vi "Process_Rect.vi"(10 "Image to process":T2, 11 "Difference image":T2) -> (0 "Target Dist":dbl, 1 "Vertical Angle":dbl, 2 "Horizontal Angle":dbl, 3 "Processed Image Out":T2, 4 "Bounding Rect":T1, 5 "Found Target":bool)   [LabVIEW 2012]
uses:
  <vilib>/vision/Image Controls.llb/IMAQ Image.ctl
  <vilib>/vision/NI_Vision_Development_Module.lvlib
panel:
  in  "Vertical Angle Offset":dbl=4.39
  out "dt 2":u32
  out "dt 1":u32
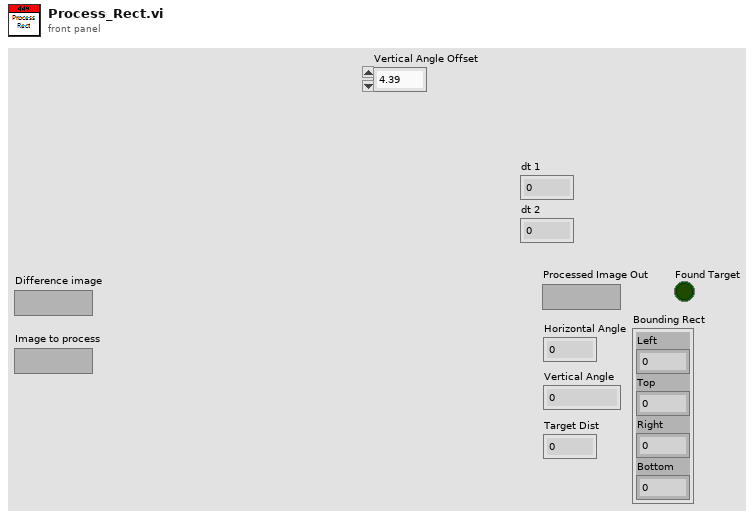
[diagram p1: front panel]
types:
  T1 = cluster{"Left":dbl, "Top":dbl, "Right":dbl, "Bottom":dbl}
  T2 = typedef "IMAQ Image.ctl" = refnum<image>
  T3 = cluster{"Area":dbl, "Number of Holes":dbl, "Bounding Rect":cluster{"Left":dbl, "Top":dbl, "Right":dbl, "Bottom":dbl}, "Center of Mass":cluster{"X":dbl, "Y":dbl}, "Orientation":dbl, "Dimensions":cluster{"Width":dbl, "Height":dbl}}[]
  T4 = cluster{"Area":dbl, "Number of Holes":dbl, "Bounding Rect":cluster{"Left":dbl, "Top":dbl, "Right":dbl, "Bottom":dbl}, "Center of Mass":cluster{"X":dbl, "Y":dbl}, "Orientation":dbl, "Dimensions":cluster{"Width":dbl, "Height":dbl}}
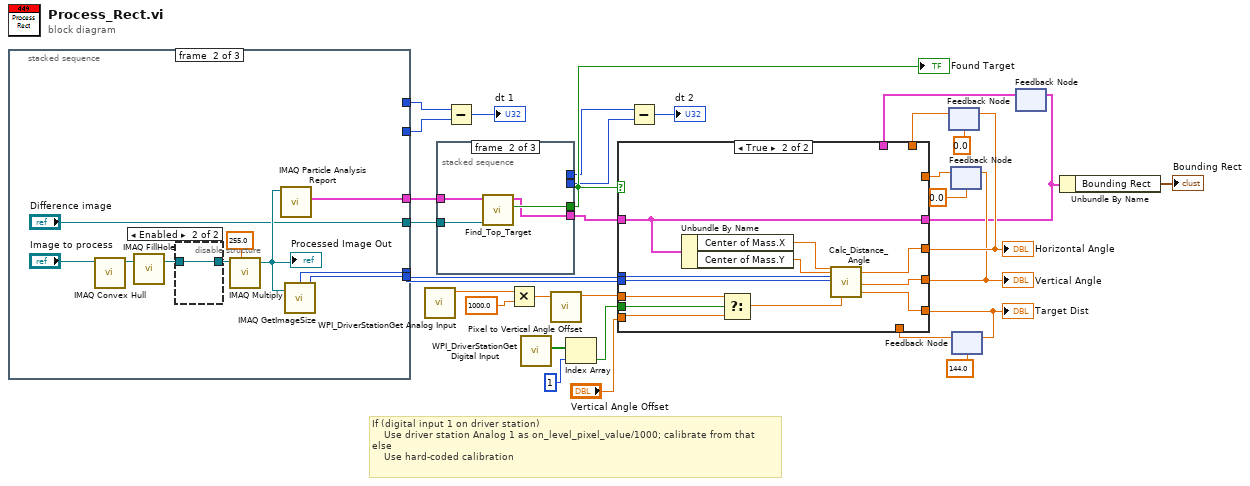
[diagram p0: block diagram]
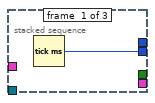
[diagram p2: hidden frame]
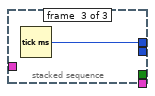
[diagram p3: hidden frame]
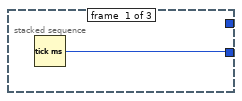
[diagram p4: hidden frame]
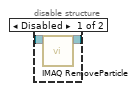
[diagram p5: hidden frame]
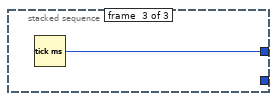
[diagram p6: hidden frame]
diagram:
  # "If (digital input 1 on driver station)\n    Use driver station Analog 1 as on_level_pixel_value/1000; calibrate from that\nelse\n    Use hard-coded calibration"
  n1 = stacked-sequence {
    tunnel: [_ w41 _] -> w32
    tunnel: [_ w40 _] -> w31
    tunnel: [_ w38 _] -> w21
    tunnel: [_ "Difference image" _] -> w18
    tunnel: [w33 _ _] -> w14
    tunnel: [_ _ w47] -> w13
    frame #0 {
      n2 = Tick Count (ms)() -> (millisecond timer value=w33:u32)
    }
    frame #1 {
      n3 = call "IMAQ Convex Hull"("Image Src"="Image to process") -> ("Image Dst Out"=w36:T2)  [unwired: 9 in, 1 out]
      n4 = call "IMAQ FillHole"("Image Src"=w36) -> ("Image Dst Out"=w37:T2)  [unwired: 5 in, 1 out]
      n5 = disable-structure shown="Enabled" {
        disable-tunnel: w37 -> [w45 w46]
        disable-tunnel: [w44 w46] -> w39
        frame Disabled {
          n6 = call "IMAQ RemoveParticle"("Image Src"=w45) -> ("Image Dst Out"=w44:T2)  [unwired: 9 in, 1 out]
        }
        frame Enabled {
        }
      }
      n7 = call "IMAQ Multiply"("Image Src A"=w39, "Constant"=sgl 255.0) -> ("Image Dst Out"=w42:T2)  [unwired: 5 in, 1 out]
      "Processed Image Out" <- w42
      n8 = call "IMAQ Particle Analysis Report"("Image"=w42) -> ("Particle Reports (Pixels)"=w38:T3)  [unwired: 5 in, 5 out]
      n9 = call "IMAQ GetImageSize"("Image"=w42) -> ("Y Resolution"=w40:i32, "X Resolution"=w41:i32)  [unwired: 3 in, 1 out]
    }
    frame #2 {
      n10 = Tick Count (ms)() -> (millisecond timer value=w47:u32)
    }
  }
  n11 = call <vilib>:"WPI_DriverStationGet Analog Input.vi"() -> ("Analog 1 (V)"=w8:dbl)  [unwired: 8 in, 3 out]
  n12 = stacked-sequence {
    tunnel: w21 -> [_ w52 _]
    tunnel: [_ w51 _] -> w20
    tunnel: [_ w50 _] -> w19
    tunnel: w18 -> [_ w49 _]
    tunnel: [w48 _ _] -> w10
    tunnel: [_ _ w53] -> w11
    frame #0 {
      n13 = Tick Count (ms)() -> (millisecond timer value=w48:u32)
    }
    frame #1 {
      n14 = call "Find_Top_Target.vi"("Difference Image"=w49, "Particle Reports (Pixels)"=w52) -> ("Found Target"=w51:bool, "Top Target"=w50:T4)  [unwired: 8 in]
    }
    frame #2 {
      n15 = Tick Count (ms)() -> (millisecond timer value=w53:u32)
    }
  }
  "Found Target" <- w20
  n16 = Subtract(x=w13, y=w14) -> (x-y=→"dt 1":u32)
  n17 = Multiply(x=w8, y=1000.0) -> (x*y=w2:dbl)
  n18 = call <vilib>:"WPI_DriverStationGet Digital Input.vi"() -> ("Driver Station Digital Input (1-8)"=w7:bool[])  [unwired: 11 in]
  n19 = call "Pixel to Vertical Angle Offset.vi"("Pixel on level with camera"=w2) -> ("Vertical Angle Offset"=w1:dbl)  [unwired: 10 in]
  n20 = Index Array(array=w7, index=1) -> (element=w5:bool)
  n21 = Subtract(x=w11, y=w10) -> (x-y=→"dt 2":u32)
  n22 = feedback #1(0.0 ("Horizontal Angle")) -> (w29:dbl)
  n23 = feedback #2(0.0 ("Horizontal Angle")) -> (w25:dbl)
  n24 = feedback #3(144.0 ("Horizontal Angle")) -> (w22:dbl)
  n25 = feedback #4() -> (w17:T4)  [unwired: 1 in]
  n26 = case shown="True" w20 {
    tunnel: w19 -> [_ w62]
    tunnel: w32 -> [_ w69]
    tunnel: w31 -> [_ w68]
    tunnel: [w57 w65] -> w28
    tunnel: [w56 w64] -> w26
    tunnel: [w55 w63] -> w23
    tunnel: w29 -> [w57 _]
    tunnel: w25 -> [w56 _]
    tunnel: w22 -> [w55 _]
    tunnel: [w54 w62] -> w16
    tunnel: w17 -> [w54 _]
    tunnel: w1 -> [_ w61]
    tunnel: w5 -> [_ w59]
    tunnel: "Vertical Angle Offset" -> [_ w58]
    frame False {
    }
    frame True {
      n27 = Unbundle By Name(w62) -> ("Center of Mass.X"=w67:dbl, "Center of Mass.Y"=w66:dbl)
      n28 = Select(t=w61, s=w59, f=w58) -> (s? t:f=w60:dbl)
      n29 = call "Calc_Distance_Angle.vi"("X Centroid"=w67, "Y Centroid"=w66, "X Res"=w69, "Y Res"=w68, "Vertical Angle Offset"=w60) -> ("Horizontal Angle"=w65:dbl, "Vertical Angle"=w64:dbl, "Target Dist"=w63:dbl)  [unwired: 19 in, 1 out]
    }
  }
  "Horizontal Angle" <- w28
  "Vertical Angle" <- w26
  "Target Dist" <- w23
  n30 = feedback-in #1(w28) -> ()
  n31 = feedback-in #2(w26) -> ()
  n32 = feedback-in #3(w23) -> ()
  n33 = feedback-in #4(w16) -> ()
  n34 = Unbundle By Name(w16) -> ("Bounding Rect"=→"Bounding Rect":T1)
